vi "Manual-Automatic Control with Saturation.vi"() -> ()   [LabVIEW 2023]
doc: "This example uses the PID Advanced VI to switch between manual and automatic control. Also, it shows how to use output range to specify the minimum and maximum value where the controller saturates the output."
uses:
  <vilib>/addons/control/pid/pid.llb/PID Advanced (DBL).vi
  <vilib>/addons/control/pid/NI_PID_pid.lvlib
panel:
  in  "SP Limit":cluster{dbl, dbl}(slide)={28.758169934640524, 80.3921568627451} scale=0.0..100.0
  in  "Auto?":bool=TRUE
  in  "SP:":dbl(slide)=54.60526315789474 scale=0.0..100.0
  in  "MV:":dbl(slide)=14.384617797820553 scale=-100.0..100.0 scale format="%#.3p"
  out "PV:":dbl(slide)=54.63887862139291 scale=0.0..100.0
  out "Output with Saturation":T1(graph)={"output"=14.384617797820553, "output high"=80.0, "output low"=0.0}
  in  "Output Controller Range":cluster{dbl, dbl}(slide)={80.0, 0.0} scale=-100.0..100.0
  out "Manual Output Range":dbl(slide)=14.384617797820553 scale=-100.0..100.0
  in  "PID gains":T2={"proportional gain (Kc)"=40.0, "integral time (Ti, min)"=0.008, "derivative time (Td, min)"=0.0} {"derivative time (Td, min)" format="%.3f"; "integral time (Ti, min)" format="%.3f"; "proportional gain (Kc)" format="%.3f"}
  in  "Stop":bool
  out "Process Variable/Setpoint":cluster{"initial PV":dbl, "SP(%)":dbl}(graph)={"initial PV"=54.63887862139291, "SP(%)"=54.60526315789474}
  # "Overview: This example uses the PID Advanced VI to switch between manual and automatic control. Also, it shows how to use output range to specify the minimum and maximum value where the controller saturates the output.\nInstructions:\n1. Run the VI and observe the Process Variable (PV) following the Setpoint (SP). However, the controller output (MV) is limited by maximum and minimum range. \n2. Change the Maximum and Minimum values and see how the controller behaves on a setpoint change.\n3. Change the setpoint to value above and below the Setpoint Limits. You will see that those values are not allowed. \n3. Click Stop to stop the VI."
  # "Change Limits below for\nOutput Range"
  # "Maximum"
  # "Minimum"
  # "Automatic"
  # "Manual"
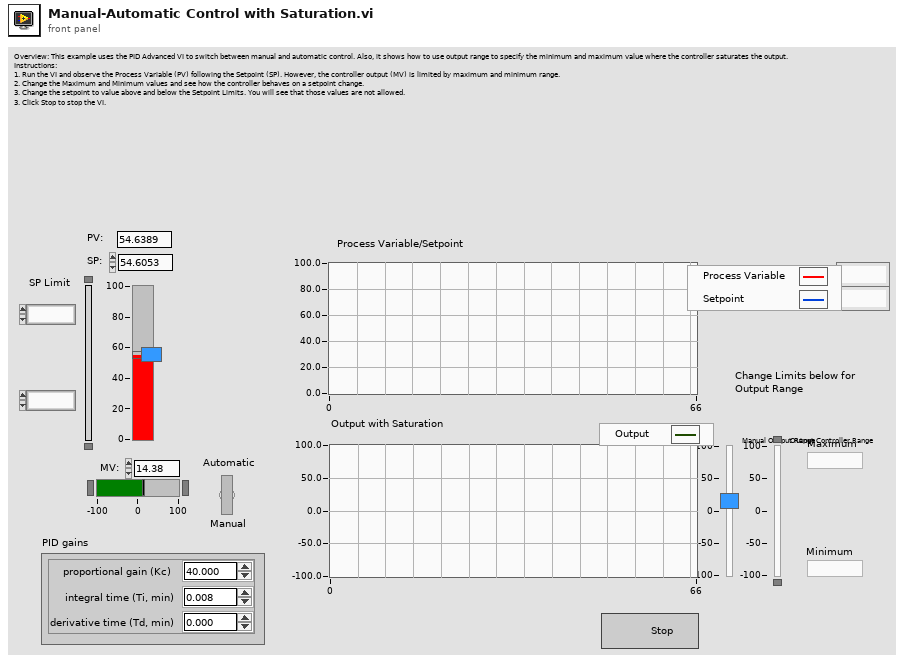
[diagram p1: front panel]
types:
  T1 = cluster{"output":dbl, "output high":dbl, "output low":dbl}
  T2 = cluster{"proportional gain (Kc)":dbl, "integral time (Ti, min)":dbl, "derivative time (Td, min)":dbl}
  T3 = cluster{"static gain":dbl, "lag (min)":dbl, "dead cycles":dbl, "load %":dbl, "deadband":dbl, "noise level %":dbl, "initial PV":dbl, "dead cycles 2":dbl}
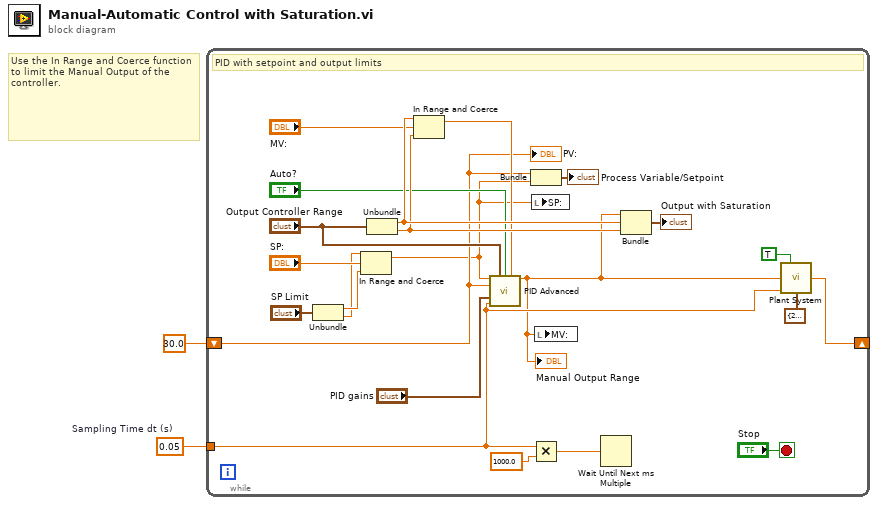
[diagram p0: block diagram]
diagram:
  w2 = 0.05  # Sampling Time dt (s)
  # "Use the In Range and Coerce function to limit the Manual Output of the controller."
  n1 = while {
    shift-left: 30.0 ("Plant Output") -> [w4]
    shift-right: [w24] -> _
    tunnel: w2 -> [w14]
    stop <- "Stop" stop-if-true
    # "PID with setpoint and output limits"
    n2 = Unbundle("SP Limit") -> (w9:dbl, w8:dbl)
    n3 = In Range and Coerce(upper limit=w8, x="SP:", lower limit=w9) -> (coerced(x)=w3:dbl)  [unwired: 1 out]
    n4 = Unbundle("Output Controller Range") -> (w19:dbl, w18:dbl)
    n5 = In Range and Coerce(upper limit=w19, x="MV:", lower limit=w18) -> (coerced(x)=w17:dbl)  [unwired: 1 out]
    n6 = call-poly <vilib>:"PID Advanced.vi"("setpoint"=w3, "output range"="Output Controller Range", "auto? (T)"="Auto?", "manual control"=w17, "process variable"=w4, "PID gains"="PID gains", "dt (s)"=w14) -> ("output"=w12:dbl)  [unwired: 7 in, 1 out]
    "Manual Output Range" <- w12
    n7 = Bundle("Plant Output"=w4, "SP:"=w3) -> (→"Process Variable/Setpoint":cluster{"Plant Output":dbl, "SP:":dbl})  [unwired: 1 in]
    n8 = Multiply(x=w14, y=1000.0) -> (x*y=w5:dbl)
    n9 = local write "SP:"(w3) -> ()
    n10 = local write "MV:"(w12) -> ()
    n11 = Wait Until Next ms Multiple(millisecond multiple=w5) -> ()  [unwired: 1 out]
    n12 = Bundle("output"=w12, w19, w18) -> (→"Output with Saturation":cluster{"output":dbl, dbl, dbl})  [unwired: 1 in]
    n13 = call "Plant System.vi"("Integrator ?"=TRUE, "Plant Input"=w12, "dt (s)"=w14, "process parameters"=T3 {"static gain"=2.5, "lag (min)"=18.0, "dead cycles"=0.0, "load %"=40.0, "deadband"=1.0, "noise level %"=0.25, "initial PV"=30.0, "dead cycles 2"=0.0} ("Process Parameters")) -> ("Plant Output"=w24:dbl)  [unwired: 11 in]
    "PV:" <- w4
  }
